vi "_ RT Read XML Method.vi"(4 "error in":errorcluster, 7 "XML String":string="<Method>\n1    0    30\n<Experiment>\n1 0 0 60000 1000 100 1 0\n<LensTable Row=\"0\"> \n</LensTable>\n<Mass Range>\n100 500 5 81 1   1\n<ParamTable Row=\"0\">\n</ParamTable>\n</Mass Range>\n</Experiment>\n</Method>") -> (0 "error out":errorcluster, 2 "Lens":T1[](array[typedef]) {"Value" format="%#.6g"}, 3 "Server Method":T2 {"Expt"."Mass Range"."Res" items=["High/High", "Medium/Medium", "Low/Low", "High/Medium", "High/Low", "Medium/High", "Medium/Low", "Low/High", "Low/Medium"]})   [LabVIEW 2015]
uses:
  Type/_Server Method.ctl
  Type/_XML Expt.ctl
  Type/_XML Lens.ctl
  Type/_Mass Range Property.ctl
  Type/_Mass Range Parameters.ctl
  Type/_RT Res Type.ctl
  Type/_RT Active Ch.ctl
  Type/_XML Type.ctl
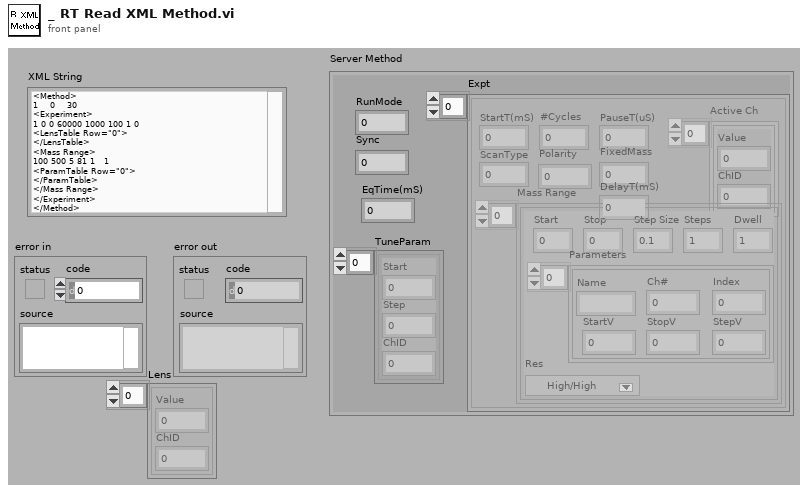
[diagram p1: front panel]
types:
  T1 = typedef "_XML Lens.ctl" = cluster{"Value":dbl, "ChID":u8}
  T2 = typedef "_Server Method.ctl" = cluster{"RunMode":i32, "Sync":u8, "Expt":T3[], "EqTime(mS)":i32, "TuneParam":T7[]}
  T3 = typedef "_XML Expt.ctl" = cluster{"StartT(mS)":i32, "#Cycles":i32, "PauseT(uS)":i32, "ScanType":i32, "Polarity":u8, "FixedMass":dbl, "DelayT(mS)":i32, "Active Ch":T1[], "Mass Range":T4[]}
  T4 = typedef "_Mass Range Property.ctl" = cluster{"Start":dbl, "Stop":dbl, "Step Size":dbl, "Steps":i32, "Dwell":dbl, "Parameters":T5[], "Res":T6}
  T5 = typedef "_Mass Range Parameters.ctl" = cluster{"Name":string, "Ch#":u8, "StartV":dbl, "StopV":dbl, "StepV":dbl, "Index":u8}
  T6 = typedef "_RT Res Type.ctl" = u16
  T7 = typedef "_RT Active Ch.ctl" = cluster{"Start":i32, "Step":i32, "ChID":i32}
  T8 = typedef "_XML Type.ctl" = enum16{"Configuration", "ConTable", "Method", "Experiment", "Mass Range", "Table", "LensTable", "ParamTable", "TuneParam", "MetParam", "MassRange", "LCMethod", "LCMethodFile", "RackType", "Vial", "PlatePos", "InjVol"}
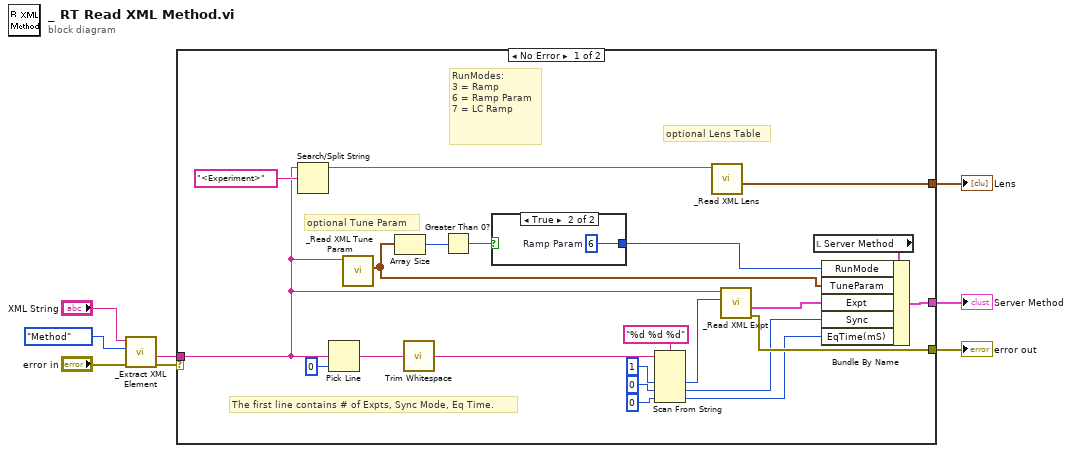
[diagram p0: block diagram]
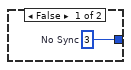
[diagram p2: hidden frame]
diagram:
  n1 = call "_Extract XML Element.vi"("error in"="error in", "XML Type"=_XML_Type."Method", "XML String"="XML String") -> ("error out"=w7:errorcluster, "Element"=w6:string)  [unwired: 3 out]
  n2 = case shown="No Error" w7 {
    selector: w7 -> [_ w33]
    tunnel: [w28 w33] -> w3
    tunnel: w6 -> [w13 _]
    tunnel: [w12 _] -> w2
    tunnel: [w11 _] -> w1
    frame No Error {
      # "RunModes:\n3 = Ramp\n6 = Ramp Param\n7 = LC Ramp"
      # "optional Tune Param"
      # "optional Lens Table"
      # "The first line contains # of Expts, Sync Mode, Eq Time."
      n3 = Search/Split String(string=w13, search string/char (-)="<Experiment>") -> (substring before match=w17:string)  [unwired: 3 out]
      n4 = Pick Line(multi-line string=w13, line index=0) -> (output string=w30:string)  [unwired: 1 out]
      n5 = call "_Read XML Tune Param.vi"("XML String"=w13) -> ("TuneParam"=w14:T7[])  [unwired: 1 in, 5 out]
      n6 = Array Size(array=w14) -> (size(s)=w16:i32)
      n7 = call <vilib>:"Trim Whitespace.vi"("string"=w30) -> ("trimmed string"=w27:string)  [unwired: 1 in]
      n8 = Greater Than 0?(x=w16) -> (x > 0?=w15:bool)
      n9 = case shown="True" w15 {
        tunnel: [w31 w32] -> w22
        frame False {
          w31 = 3  # No Sync
        }
        frame True {
          w32 = 6  # Ramp Param
        }
      }
      n10 = Scan From String(format string="%d %d %d", input string=w27, default 1=1 ("Ch#"), default 2=u8 0 ("Ch#"), default 3=0 ("Ch#")) -> (output 1=w26:i32, output 2=w10:u8, output 3=w9:i32)  [unwired: 2 in, 3 out]
      n11 = call "_Read XML Lens.vi"("XML String"=w17) -> ("Lens"=w11:T1[])  [unwired: 1 in, 5 out]
      n12 = call "_Read XML Expt.vi"("# of Expts"=w26, "XML String"=w13) -> ("error out"=w28:errorcluster, "Expt"=w18:T3[])  [unwired: 1 in, 3 out]
      n13 = local read "Server Method"() -> (w23:T2)
      n14 = Bundle By Name(cluster=w23, "RunMode"=w22, "TuneParam"=w14, "Expt"=w18, "Sync"=w10, "EqTime(mS)"=w9) -> (w12:T2)
    }
    frame Error {
    }
  }
  "error out" <- w3
  "Server Method" <- w2
  "Lens" <- w1
